vi "Save Library Documentation.vi"(9 "New Description":string, 10 "DQMH Modules Info In":T1, 11 "Library in":refnum<vi>) -> (0 "error out":errorcluster, 2 "DQMH Modules Info Out":T1, 3 "Lib out":refnum<vi>)   [LabVIEW 2019, in "Panther Dashboard.lvlib"]
uses:
  Panther Dashboard.lvlib
  Module type--enum.ctl
  DQMH Modules Info--cluster.ctl
  Project References--cluster.ctl
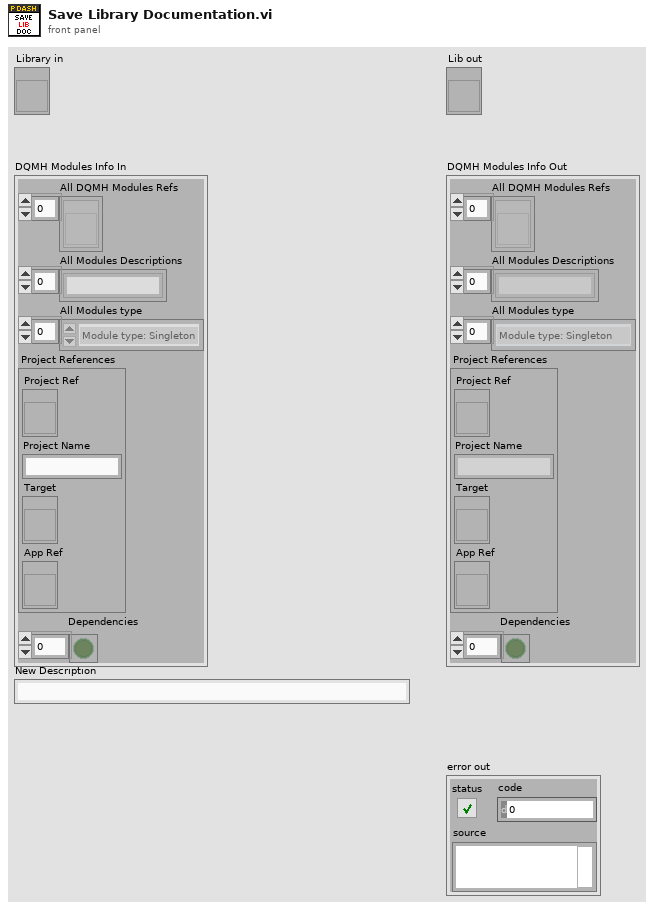
[diagram p1: front panel]
types:
  T1 = typedef "Panther Dashboard.lvlib/DQMH Modules Info--cluster.ctl" = cluster{"All DQMH Modules Refs":refnum<vi>[], "All Modules Descriptions":string[], "All Modules type":T2[], "Project References":T3, "Dependencies":bool[]}
  T2 = typedef "Panther Dashboard.lvlib/Module type--enum.ctl" = enum16{"Module type: Singleton", "Module type: Cloneable"}
  T3 = typedef "Panther Dashboard.lvlib/Project References--cluster.ctl" = cluster{"Project Ref":refnum<vi>, "Project Name":string, "Target":refnum<vi>, "App Ref":refnum<vi>}
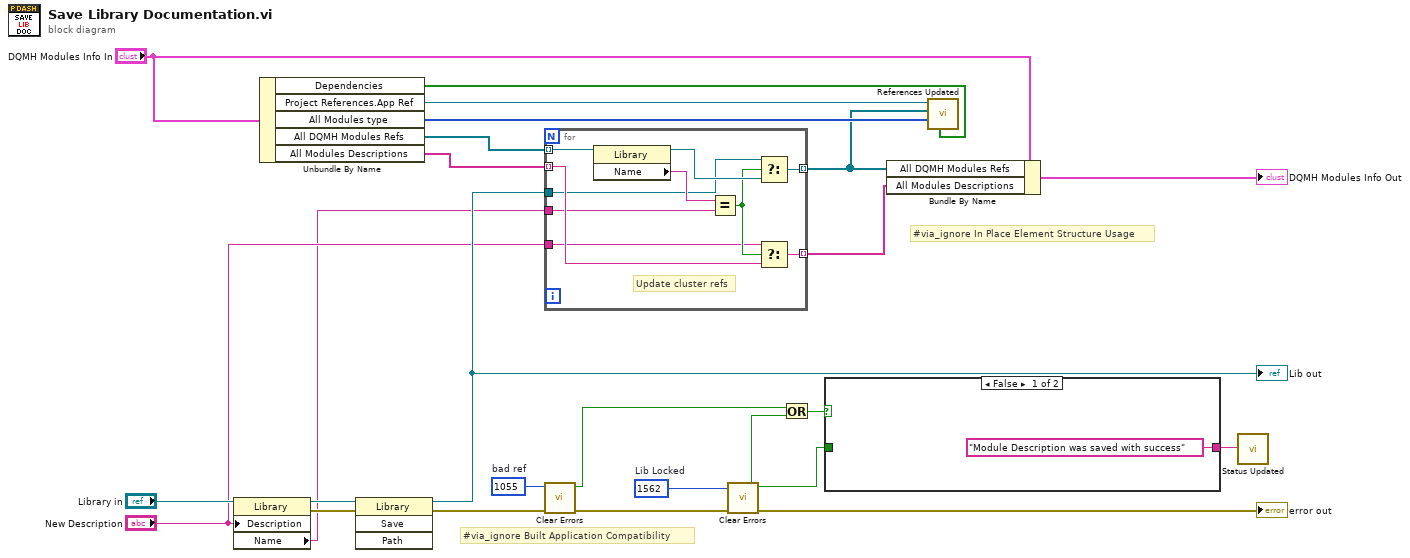
[diagram p0: block diagram]
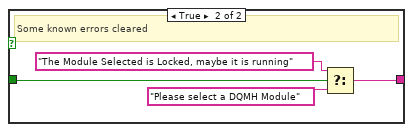
[diagram p2: hidden frame]
diagram:
  w8 = 1562  # Lib Locked
  w9 = 1055  # bad ref
  # "#via_ignore Built Application Compatibility"
  # "#via_ignore In Place Element Structure Usage"
  n1 = property class="Library"(reference="Library in", "Description"="New Description") -> (reference out=w18:refnum<vi>, error out=w24:errorcluster, "Name"=w11:string)  [unwired: 1 in]
  n2 = Unbundle By Name("DQMH Modules Info In") -> ("Dependencies"=w1:bool[], "Project References.App Ref"=w3:refnum<vi>, "All Modules type"=w4:T2[], "All DQMH Modules Refs"=w19:refnum<vi>[], "All Modules Descriptions"=w14:string[])
  n3 = invoke class="Library" method="Save"(reference=w18, error in=w24) -> (reference out=w15:refnum<vi>, error out=w23:errorcluster)  [unwired: 2 in, 2 out]
  "Lib out" <- w15
  n4 = for {
    tunnel: w19 -> [w34] mode=indexing
    tunnel: [w31] -> w2 mode=indexing
    tunnel: w15 -> [w25]
    tunnel: w14 -> [w29] mode=indexing
    tunnel: [w28] -> w13 mode=indexing
    tunnel: "New Description" -> [w27]
    tunnel: w11 -> [w26]
    # "Update cluster refs"
    n5 = property class="Library"(reference=w34) -> (reference out=w32:refnum<vi>, "Name"=w33:string)  [unwired: 1 in, 1 out]
    n6 = Equal?(x=w33, y=w26) -> (x = y?=w30:bool)
    n7 = Select(t=w25, s=w30, f=w32) -> (s? t:f=w31:refnum<vi>)
    n8 = Select(t=w27, s=w30, f=w29) -> (s? t:f=w28:string)
  }
  n9 = call <vilib>:"Clear Errors.vi"("error in (no error)"=w23, "specific error code to clear (0: all)"=w9) -> ("error out"=w22:errorcluster, "specific error cleared?"=w10:bool)  [unwired: 4 in]
  n10 = call <vilib>:"Clear Errors.vi"("error in (no error)"=w22, "specific error code to clear (0: all)"=w8) -> ("error out"=→"error out":errorcluster, "specific error cleared?"=w6:bool)  [unwired: 4 in]
  n11 = Or(x=w10, y=w6) -> (x .or. y?=w7:bool)
  n12 = case shown="False" w7 {
    tunnel: w6 -> [_ w39]
    tunnel: ["Module Description was saved with success" ("Status") w36] -> w5
    frame False {
    }
    frame True {
      # "Some known errors cleared"
      n13 = Select(t="The Module Selected is Locked, maybe it is running" ("Status"), s=w39, f="Please select a DQMH Module" ("Status")) -> (s? t:f=w36:string)
    }
  }
  n14 = Bundle By Name(cluster="DQMH Modules Info In", "All DQMH Modules Refs"=w2, "All Modules Descriptions"=w13) -> (→"DQMH Modules Info Out":T1)
  n15 = call "References Updated.vi"("Dependencies"=w1, "Modules Types"=w4, "Modules"=w2, "Application Instance"=w3) -> ()  [unwired: 7 in, 1 out]
  n16 = call "Status Updated.vi"("Status"=w5) -> ()  [unwired: 10 in, 1 out]
